vi "ModifyHTML_+CreatedTempPath_xPNG.vi"(6 "Identifying_String":string="img src=\"", 8 "error in (no error)":errorcluster, 9 "Dencrypted text":string, 10 "SubFolderName":string, 11 "Folder_Mgmt":refnum<class "Folder_Mgmt.lvclass">) -> (0 "error out":errorcluster, 1 "ModifyedHTML":string, 2 "TemporaryFiles":path[](array[path]), 3 "Folder_Mgmt 2":refnum<class "Folder_Mgmt.lvclass">)   [LabVIEW 2016, in "Folder_Mgmt.lvclass"]
uses:
  Folder_Mgmt.lvclass
  Folder_Mgmt.lvclass/Folder_Mgmt.ctl
panel:
  out "before substring":string
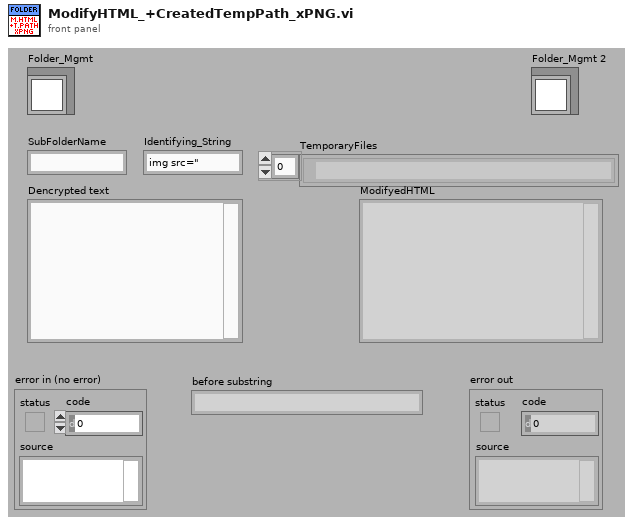
[diagram p1: front panel]
types:
  T1 = enum16{"open", "replace", "create", "open or create", "replace or create", "replace or create with confirmation"}
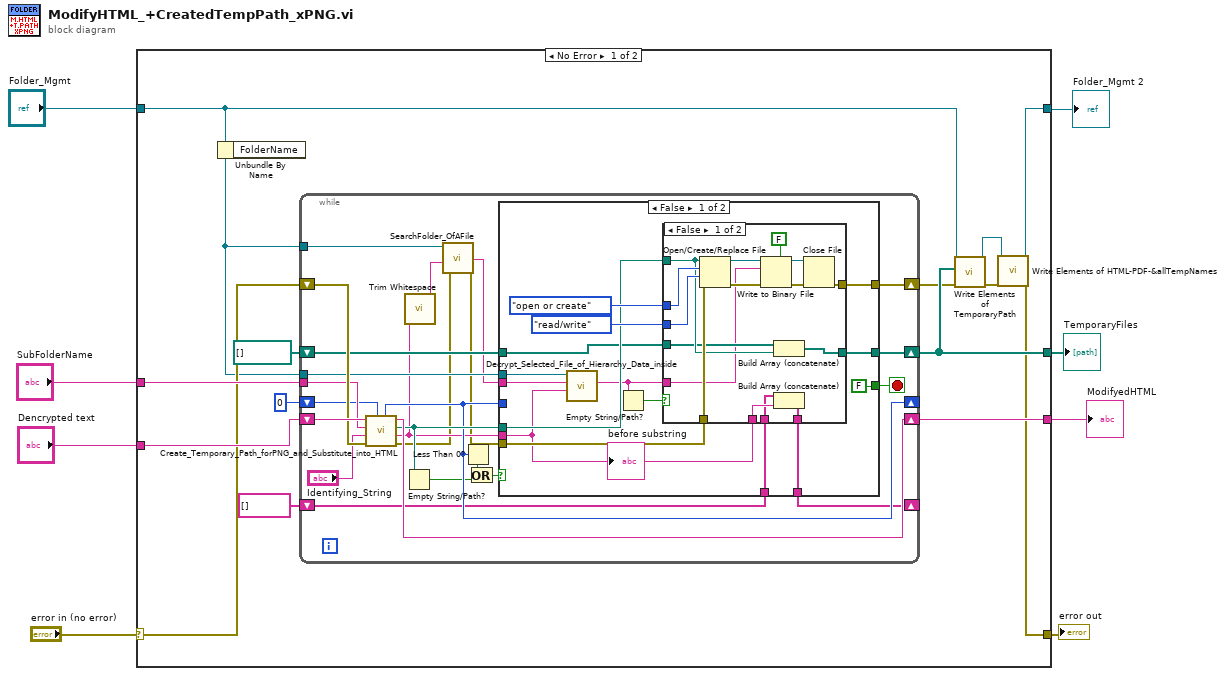
[diagram p0: block diagram]
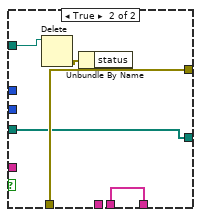
[diagram p2: hidden frame]
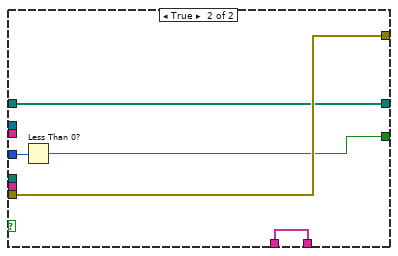
[diagram p3: hidden frame]
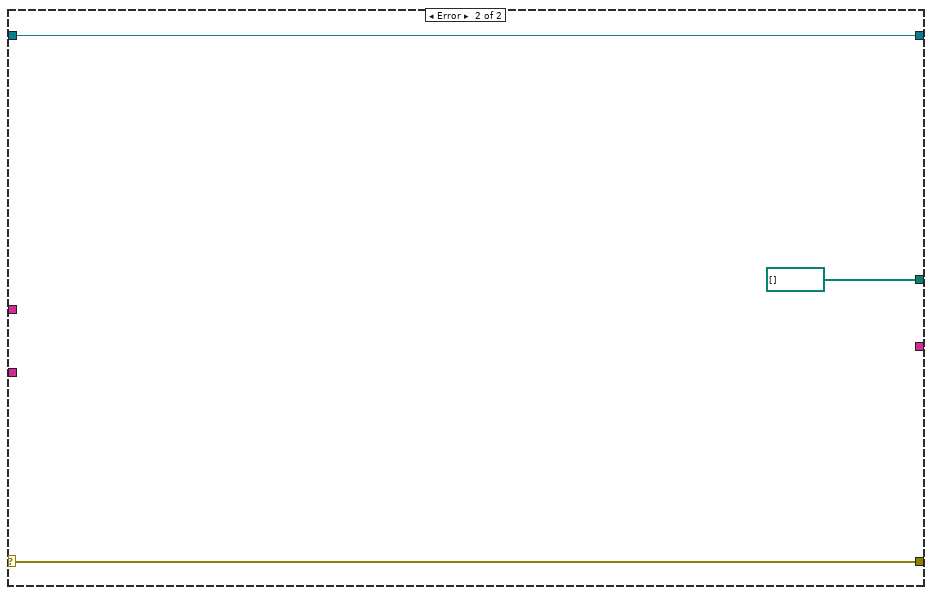
[diagram p4: hidden frame]
diagram:
  n1 = case shown="No Error" "error in (no error)" {
    selector: "error in (no error)" -> [w19 w90]
    tunnel: [w12 w90] -> w7
    tunnel: [w10 w89] -> w2
    tunnel: "Folder_Mgmt" -> [w14 w89]
    tunnel: "SubFolderName" -> [w21 _]
    tunnel: "Dencrypted text" -> [w20 _]
    tunnel: [w16 path[] []] -> w4
    tunnel: [w18 _] -> w3
    frame No Error {
      n2 = Unbundle By Name(w14) -> ()  [unwired: 1 out]
      n3 = while {
        tunnel: w14 -> [w42]
        tunnel: w21 -> [w39]
        shift-right: [w46] -> w15
        shift-left: w19 -> [w43]
        shift-right: [w44] -> w18
        shift-left: w20 -> [w45]
        shift-right: [w35] -> _
        shift-left: 0 ("offset past match") -> [w37]
        shift-right: [w40] -> w16
        shift-left: path[] [] -> [w32]
        tunnel: w14 -> [w30]
        shift-right: [w24] -> _
        shift-left: string[] [] -> [w23]
        stop <- w38 stop-if-true
        n4 = call "Create_Temporary_Path_forPNG_and_Substitute_into_HTML.vi"("offset past match"=w37, "error in (no error)"=w43, "Identifying_String"="Identifying_String", "SubFolderName"=w39, "Dencrypted text"=w45) -> ("error out"=w27:errorcluster, "PNG_fileName"=w29:string, "Temp_PATH"=w41:path, "HTML_wPathChanged"=w44:string, "offset past match"=w35:i32)  [unwired: 2 in]
        n5 = Empty String/Path?(string/path=w41) -> (empty?=w31:bool)
        n6 = call <vilib>:"Trim Whitespace.vi"("string"=w29) -> ("trimmed string"=w28:string)  [unwired: 1 in]
        n7 = call "SearchFolder_OfAFile.vi"("Folder_Mgmt out"=w30, "FileToSearch"=w28, "error in (no error)"=w27) -> ("FolderOfFile"=w25:string, "error out"=w26:errorcluster)  [unwired: 5 in, 1 out]
        n8 = Less Than 0?(x=w35) -> (x < 0?=w34:bool)
        n9 = Or(x=w34, y=w31) -> (x .or. y?=w36:bool)
        n10 = case shown="False" w36 {
          tunnel: [w59 w87] -> w46
          tunnel: w29 -> [w49 _]
          tunnel: w26 -> [w58 w87]
          tunnel: w42 -> [w57 _]
          tunnel: w25 -> [w56 _]
          tunnel: w41 -> [w55 _]
          tunnel: [w53 w86] -> w40
          tunnel: [FALSE w83] -> w38
          tunnel: w35 -> [_ w84]
          tunnel: w32 -> [w52 w86]
          tunnel: [w48 w85] -> w24
          tunnel: w23 -> [w47 w85]
          frame False {
            n11 = call-dynamic "Decrypt_Selected_File_of_Hierarchy_Data_inside.vi"("FileName"=w49, "SubFolderName"=w56, "object in"=w57) -> ("Dencrypted text"=w51:string)  [unwired: 5 in, 3 out]
            n12 = Empty String/Path?(string/path=w51) -> (empty?=w50:bool)
            n13 = case shown="False" w50 {
              tunnel: enum16{"read/write", "read-only", "write-only"}."read/write" ("access (0:read/write)") -> [w73 _]
              tunnel: T1."open or create" ("operation (0:open)") -> [w72 _]
              tunnel: [w70 w82] -> w59
              tunnel: w58 -> [w69 w82]
              tunnel: w55 -> [w68 w80]
              tunnel: [w67 w81] -> w53
              tunnel: w52 -> [w66 w81]
              tunnel: w51 -> [w65 _]
              tunnel: w49 -> [w64 _]
              tunnel: [w63 w78] -> w48
              tunnel: w47 -> [w62 w78]
              frame False {
                n14 = Open/Create/Replace File(file path (use dialog)=w68, error in=w69, operation (0:open)=w72, access (0:read/write)=w73) -> (refnum out=w74:refnum<file>, error out=w75:errorcluster)  [unwired: 2 in, 1 out]
                n15 = Write to Binary File(file (use dialog)=w74, data=w65, error in=w75, 5:FALSE ("prepend array or string size? (T)")) -> (refnum out=w77:refnum<file>, error out=w76:errorcluster)  [unwired: 2 in, 1 out]
                n16 = Build Array (concatenate)(w66, w68) -> (w67:path[])
                n17 = Build Array (concatenate)(w62, w64) -> (w63:string[])
                n18 = Close File(refnum=w77, error in=w76) -> (error out=w70:errorcluster)  [unwired: 1 out]
              }
              frame True {
                n19 = Delete(path (use dialog)=w80) -> (error out=w79:errorcluster)  [unwired: 4 in, 2 out]
                n20 = Unbundle By Name(w79) -> ()  [unwired: 1 out]
              }
            }
            "before substring" <- w49
          }
          frame True {
            n21 = Less Than 0?(x=w84) -> (x < 0?=w83:bool)
          }
        }
      }
      n22 = call "Write Elements of TemporaryPath.vi"("error in (no error)"=w15, "Paths"=w16, "Folder_Mgmt"=w14) -> ("error out"=w13:errorcluster, "Folder_Mgmt 2"=w11:refnum<class "Folder_Mgmt.lvclass">)  [unwired: 7 in]
      n23 = call "Write Elements of HTML-PDF-&allTempNames.vi"("error in (no error)"=w13, "Folder_Mgmt"=w11) -> ("error out"=w12:errorcluster, "Folder_Mgmt 2"=w10:refnum<class "Folder_Mgmt.lvclass">)  [unwired: 8 in]
    }
    frame Error {
    }
  }
  "error out" <- w7
  "TemporaryFiles" <- w4
  "ModifyedHTML" <- w3
  "Folder_Mgmt 2" <- w2
